vi "Notify State.vi"(8 "error in (no error)":errorcluster, 11 "State Machine Actor in":refnum<class "State Machine Actor.lvclass">) -> (0 "error out":errorcluster, 3 "State Machine Actor out":refnum<class "State Machine Actor.lvclass">)   [LabVIEW 2024, in "State Machine Actor.lvlib" / "State Machine Actor.lvclass"]
uses:
  State Machine Actor.lvclass
  State Machine Actor.lvclass/State Machine Actor.ctl
  C:/Users/uspoaotto/OneDrive - Oregon Tool/Desktop/working copies/stateMachineActor/src/_State Machine Actor/_State Machine Actor/_State Machine Actor.lvclass
  C:/Program Files (x86)/National Instruments/LabVIEW 2024/vi.lib/ActorFramework/Actor/Actor.lvclass
  C:/Users/uspoaotto/OneDrive - Oregon Tool/Desktop/working copies/stateMachineActor/src/State Machine Actor/State Machine Actor/State Machine Actor.lvclass
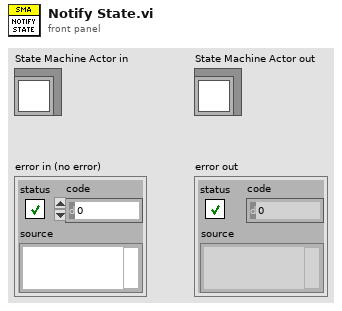
[diagram p1: front panel]
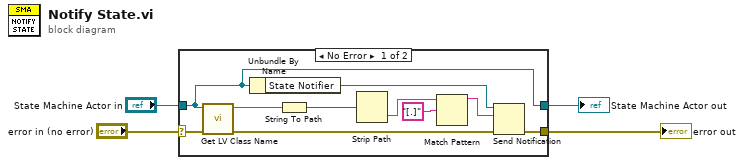
[diagram p0: block diagram]
diagram:
  n1 = case shown="No Error" "error in (no error)" {
    selector: "error in (no error)" -> [w7 w16]
    tunnel: [w6 w16] -> w3
    tunnel: [w10 w15] -> w1
    tunnel: "State Machine Actor in" -> [w10 w15]
    frame No Error {
      n2 = call <vilib>:"Get LV Class Name.vi"("error in (no error)"=w7, "object"=w10) -> ("error out"=w8:errorcluster, "class name"=w13:string)  [unwired: 8 in]
      n3 = Unbundle By Name(w10) -> ("State Notifier"=w14:refnum<notifier>)
      n4 = String To Path(string=w13) -> (path=w12:path)
      n5 = Strip Path(path=w12) -> (name=w9:string)  [unwired: 1 out]
      n6 = Match Pattern(string=w9, regular expression="[.]") -> (before substring=w5:string)  [unwired: 1 in, 3 out]
      n7 = Send Notification(notification=w5, notifier=w14, error in (no error)=w8) -> (error out=w6:errorcluster)  [unwired: 1 out]
    }
    frame Error {
    }
  }
  "error out" <- w3
  "State Machine Actor out" <- w1
